vi "Err.vi"(1 "error in":errorcluster) -> (0 "error out":errorcluster)   [LabVIEW 2010]
uses:
  <vilib>/Utility/file.llb/Write To Spreadsheet File (string).vi
  <vilib>/Utility/error.llb/DialogType.ctl
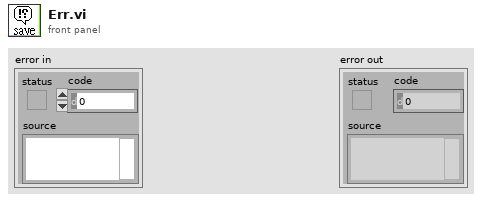
[diagram p1: front panel]
types:
  T1 = typedef "DialogType.ctl" = u16
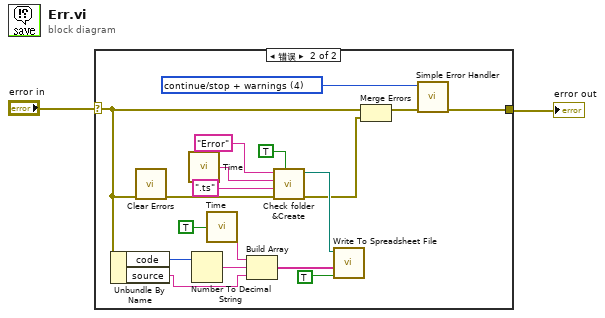
[diagram p0: block diagram]
diagram:
  n1 = case shown="错误" "error in" {
    selector: "error in" -> [w3 w7]
    tunnel: [w3 w14] -> w1
    frame No Error {
    }
    frame Error {
      w13 = T1 4 items=["no dialog", "OK message", "continue or stop message", "OK message + warnings", "continue/stop + warnings"] ("type of dialog (OK msg:1)")
      n2 = Unbundle By Name(w7) -> ("code"=w16:i32, "source"=w15:string)
      n3 = call <vilib>:"Clear Errors.vi"("error in (no error)"=w7) -> ("error out"=w6:errorcluster)  [unwired: 6 in]
      n4 = call "Time.vi"() -> ("Time"=w10:string)  [unwired: 1 in]
      n5 = Number To Decimal String(number=w16) -> (decimal integer string=w19:string)  [unwired: 1 in]
      n6 = call "Time.vi"("format"=TRUE) -> ("Time"=w20:string)
      n7 = Build Array(w20, w19, w15) -> (w18:string[])
      n8 = call "Check folder &Create.vi"("Boolean"=TRUE, "error in (no error)"=w6, "pattern"=".ts", "file name"=w10, "folder name"="Error") -> ("error out"=w4:errorcluster, "build path"=w8:path)  [unwired: 5 in]
      n9 = call-poly <vilib>:"Write To Spreadsheet File.vi"("append to file? (new file:F)"=TRUE, "1D data"=w18, "file path (dialog if empty)"=w8) -> ()  [unwired: 5 in, 1 out]
      n10 = Merge Errors(w7, w4) -> (w5:errorcluster)
      n11 = call <vilib>:"Simple Error Handler.vi"("type of dialog (OK msg:1)"=w13, "error in (no error)"=w5) -> ("error out"=w14:errorcluster)  [unwired: 3 in, 4 out]
    }
  }
  "error out" <- w1
